vi "random.vi"(9 "min":i32, 10 "max":i32) -> (2 "random":i32)   [LabVIEW 2017, in "ThirdPartyYoutubeClass.lvclass"]
uses:
  ThirdPartyYoutubeClass.lvclass
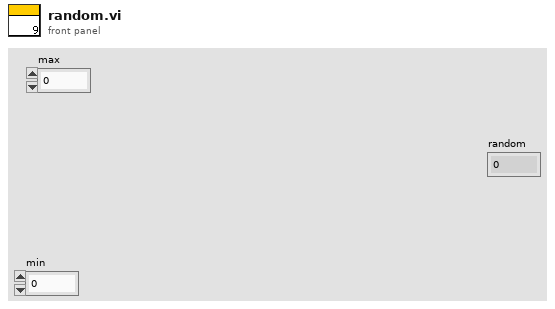
[diagram p1: front panel]
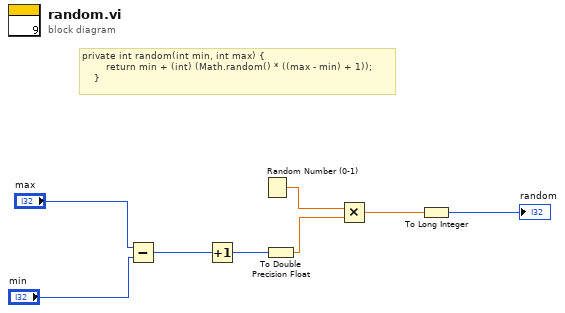
[diagram p0: block diagram]
diagram:
  # "private int random(int min, int max) {\n        return min + (int) (Math.random() * ((max - min) + 1));\n    }"
  n1 = Subtract(x="max", y="min") -> (x-y=w6:i32)
  n2 = Increment(x=w6) -> (x+1=w4:i32)
  n3 = Random Number (0-1)() -> (number: 0 to 1=w5:dbl)
  n4 = To Double Precision Float(number=w4) -> (double precision float=w3:dbl)
  n5 = Multiply(x=w5, y=w3) -> (x*y=w2:dbl)
  n6 = To Long Integer(number=w2) -> (32bit integer=→"random":i32)
